vi "GlobalCollectDataRefOperate.vi"(7 "ChannelNbr":u8, 8 "error in (no error)":errorcluster, 9 "DatIn":dbl[][](array[numeric]), 10 "operation":T1, 11 "attributes ref":T2) -> (0 "error out":errorcluster, 1 "SignalDatOut":dbl[][](array[numeric]), 2 "Update":bool)   [LabVIEW 2020, in "DAQ_Base.lvclass"]
doc: "---------------------------------------------------------------\nJKI State Machine Objects™\nhttp://jki.net/state-machine-objects/\nCopyright (C) 2005-2015, JKI <info@jki.net>\nALL RIGHTS RESERVEDJKI State Machine Objects (SMO) 1.0.0.5\nJKI - JKI\nCopyright (c) 2016, JKI"
uses:
  DAQ_Base.lvclass
  utils/ObjectAttributesRef.ctl
  protected/ObjectAttributes.ctl
  protected/DAQSettings.ctl
  protected/SampleSettings.ctl
  protected/AI_ChannelSettings.ctl
  protected/AO_ChannelSettings.ctl
  protected/Cnt_ChannelSettings.ctl
  protected/DataCollector.ctl
  GlobalData_operation.ctl
panel:
  # "For instructions on how to use the JKI State Machine Objects, examples and video tutorials, visit:\nhttp://jki.net/state-machine-objects/\n\nJKI State Machine Objects™\nhttp://jki.net/state-machine-objects/\nCopyright (C) 2005-2015, JKI <info@jki.net>\nALL RIGHTS RESERVED"
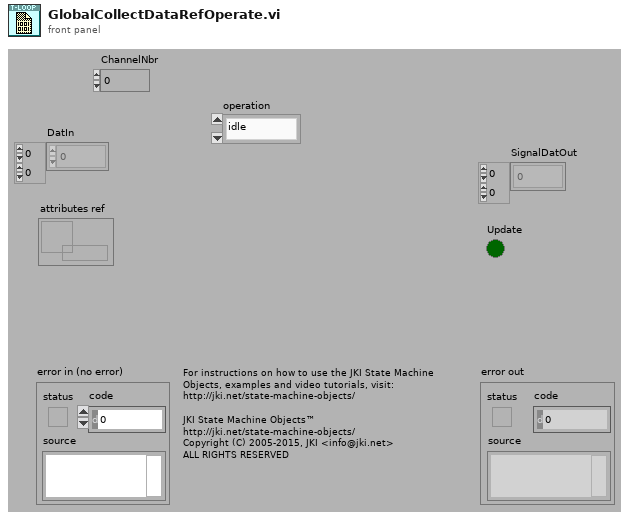
[diagram p1: front panel]
types:
  T1 = typedef "GlobalData_operation.ctl" = enum16{"idle", "read", "write", "clear", "init", "destroy"}
  T2 = typedef "DAQ_Base.lvclass/ObjectAttributesRef.ctl" = refnum<data-value>
  T3 = typedef "DAQ_Base.lvclass/DataCollector.ctl" = cluster{"DataCollectArry":dbl[][], "Update":bool}
  T4 = cluster{"DataCollectArry":dbl[][], "Update":bool}
  T5 = typedef "DAQ_Base.lvclass/ObjectAttributes.ctl" = cluster{"MyAttribute":dbl, "RootPath":path, "DAQSettings":T6, "DaqCollector":cluster{"CollectorChannelEnable":bool[], "CollectDataQueue":refnum<queue>, "ArryDataCollectorChannel":T3[], "RealTimeValues":dbl[]}}
  T6 = typedef "DAQ_Base.lvclass/DAQSettings.ctl" = cluster{"SampleSettings":T7, "AI_ChannelSettings":T8, "AO_ChannelSettings":T10, "Cnt_ChannelSettings":T11}
  T7 = typedef "DAQ_Base.lvclass/SampleSettings.ctl" = cluster{"samples per channel":i32, "SampleRate":dbl, "TansMaxLength":dbl, "ReadTimeOut":dbl, "时钟源":tag}
  T8 = typedef "DAQ_Base.lvclass/AI_ChannelSettings.ctl" = cluster{"AI_SettingsArry":cluster{"DeviceName":tag, "physical channels":tag, "AssignName":string, "输入信号类型":T9, "Max_value":dbl, "Min_value":dbl, "单位":i32, "shunt resistor location":i32, "external shunt resistor value":dbl, "标定系数":cluster{"Scale":dbl, "Offset":dbl}}[]}
  T9 = typedef "AI信号类型.ctl" = i32
  T10 = typedef "DAQ_Base.lvclass/AO_ChannelSettings.ctl" = cluster{"布尔":bool}
  T11 = typedef "DAQ_Base.lvclass/Cnt_ChannelSettings.ctl" = cluster{"Cnt_ChannelSettings":cluster{"类型":enum16{"Linear", "Rotate"}, "CounterNbr":tag, "AssignName":string, "单位":u16, "decoding type":u16, "PPR_DistancePerPulse":dbl, "Initial Position ":dbl, "z index enable":bool, "z index phase":i32, "source":tag}[]}
  T12 = cluster{"DataCollectArry":dbl[][], "Update":bool}[]
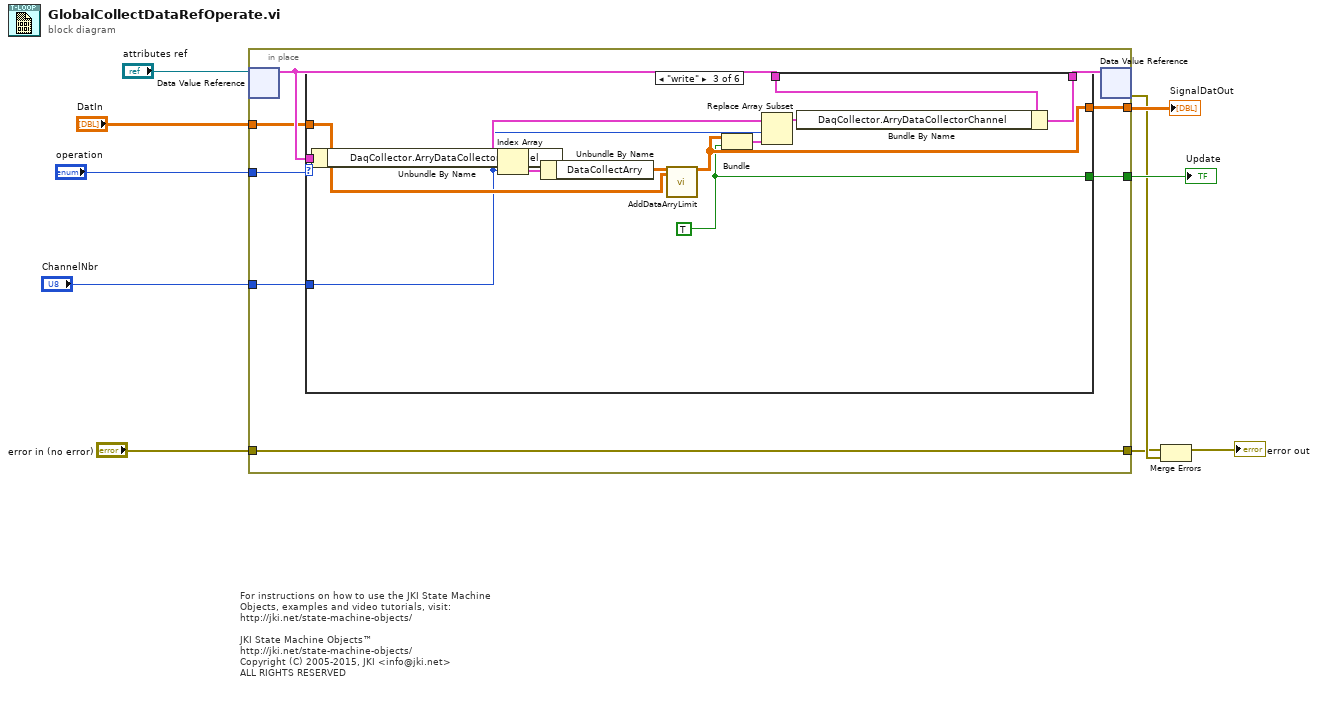
[diagram p0: block diagram]
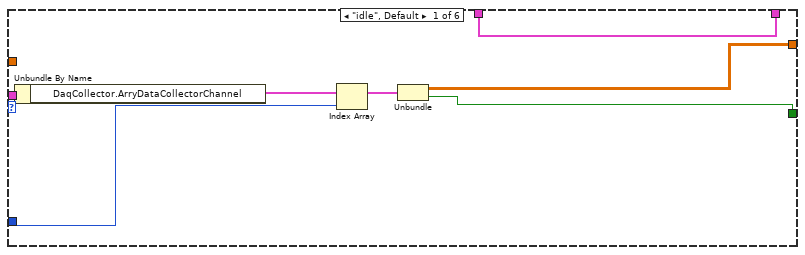
[diagram p2: hidden frame]
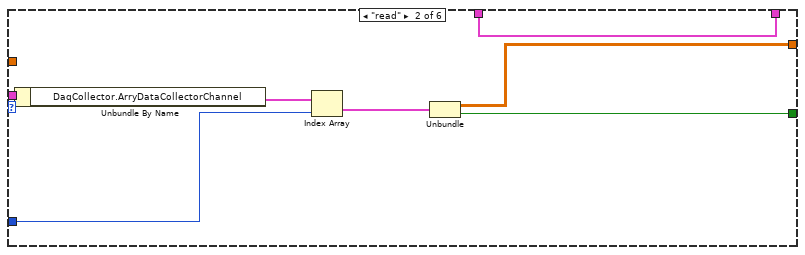
[diagram p3: hidden frame]
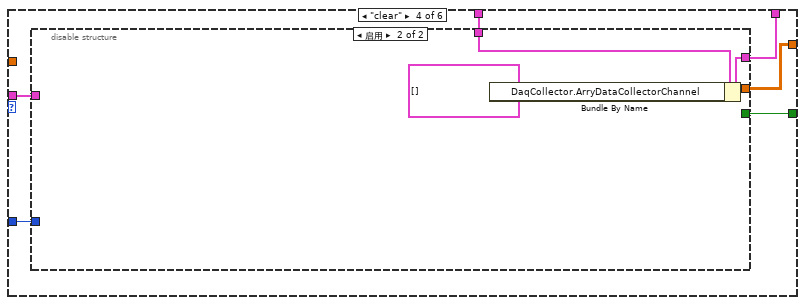
[diagram p4: hidden frame]
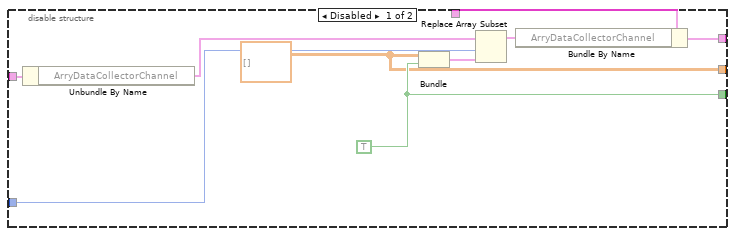
[diagram p5: hidden frame]
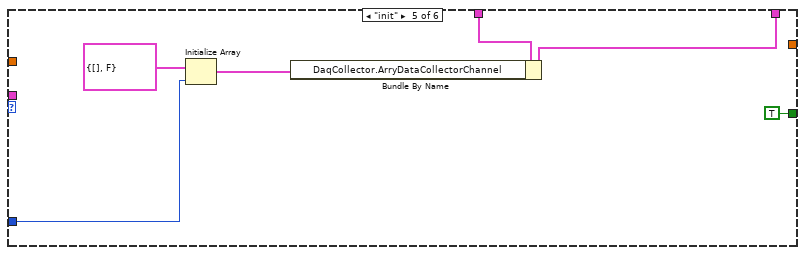
[diagram p6: hidden frame]
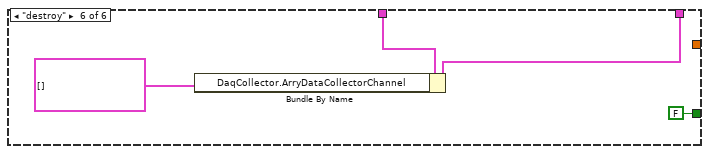
[diagram p7: hidden frame]
diagram:
  # "For instructions on how to use the JKI State Machine Objects, examples and video tutorials, visit:\nhttp://jki.net/state-machine-objects/\n\nJKI State Machine Objects™\nhttp://jki.net/state-machine-objects/\nCopyright (C) 2005-2015, JKI <info@jki.net>\nALL RIGHTS RESERVED"
  n1 = in-place {
    in-place-border: "error in (no error)" -> [w18]
    in-place-border: [w18] -> w1
    in-place-border: [w17] -> w6
    in-place-border: "operation" -> [w16]
    in-place-border: [w15] -> w8
    in-place-border: "DatIn" -> [w12]
    in-place-border: "ChannelNbr" -> [w11]
    n2 = in-place-dvr #1("attributes ref") -> (w14:T5)  [unwired: 1 out]
    n3 = case shown="\"write\"" w16 {
      tunnel: [w20 w27 w38 w45 _ _] -> w17
      tunnel: w14 -> [w22 w30 w44 w50 _ _]
      tunnel: [w19 w26 w37 w47 TRUE ("Update") FALSE ("Update")] -> w15
      tunnel: w14 -> [w25 w32 w43 w49 w68 w72]
      tunnel: [w25 w32 w42 w48 w67 w71] -> w13
      tunnel: w12 -> [_ _ w41 _ _ _]
      tunnel: w11 -> [w21 w29 w35 w46 w64 _]
      frame "idle", Default {
        n4 = Unbundle By Name(w22) -> ("DaqCollector.ArryDataCollectorChannel"=w24:T3[])
        n5 = Index Array(array=w24, index=w21) -> (element=w23:T3)
        n6 = Unbundle(w23) -> ("DataCollectArry"=w20:dbl[][], "Update"=w19:bool)
      }
      frame "read" {
        n7 = Unbundle By Name(w30) -> ("DaqCollector.ArryDataCollectorChannel"=w31:T3[])
        n8 = Index Array(array=w31, index=w29) -> (element=w28:T3)
        n9 = Unbundle(w28) -> ("DataCollectArry"=w27:dbl[][], "Update"=w26:bool)
      }
      frame "write" {
        w37 = TRUE
        n10 = Unbundle By Name(w44) -> ("DaqCollector.ArryDataCollectorChannel"=w36:T3[])
        n11 = Index Array(array=w36, index=w35) -> (element=w40:T3)
        n12 = Unbundle By Name(w40) -> ("DataCollectArry"=w39:dbl[][])
        n13 = call "AddDataArryLimit.vi"("MainDataArryIn"=w39, "SubDataArry"=w41) -> ("输出数组"=w38:dbl[][])  [unwired: 17 in]
        n14 = Bundle("输出数组"=w38, w37) -> (w34:cluster{"输出数组":dbl[][], bool})  [unwired: 1 in]
        n15 = Replace Array Subset(array=w36, new element=w34, index=w35) -> (w33:T3[])
        n16 = Bundle By Name(cluster=w43, "DaqCollector.ArryDataCollectorChannel"=w33) -> (w42:T5)
      }
      frame "clear" {
        n17 = disable-structure shown="启用" {
          disable-tunnel: w50 -> [w59 _]
          disable-tunnel: w49 -> [w58 w62]
          disable-tunnel: [w57 w61] -> w48
          disable-tunnel: [w56 _] -> w47
          disable-tunnel: w46 -> [w54 _]
          disable-tunnel: [w51 _] -> w45
          frame Disabled {
            w51 = dbl[][] [] ("DatIn")
            w56 = TRUE
            n18 = Unbundle By Name(w59) -> ("ArryDataCollectorChannel"=w55:T3[])
            n19 = Bundle("DatIn"=w51, w56) -> (w53:cluster{"DatIn":dbl[][], bool})  [unwired: 1 in]
            n20 = Replace Array Subset(array=w55, new element=w53, index=w54) -> (w52:T3[])
            n21 = Bundle By Name(cluster=w58, "ArryDataCollectorChannel"=w52) -> (w57:T5)
          }
          frame Enabled {
            n22 = Bundle By Name(cluster=w62, "DaqCollector.ArryDataCollectorChannel"=T3[] [] ("ArryDataCollectorChannel")) -> (w61:T5)
          }
        }
      }
      frame "init" {
        n23 = Initialize Array(T4 {"DataCollectArry"=[], "Update"=FALSE} ("DataCollectorChannel"), w64) -> (w63:T12)
        n24 = Bundle By Name(cluster=w68, "DaqCollector.ArryDataCollectorChannel"=w63) -> (w67:T5)
      }
      frame "destroy" {
        n25 = Bundle By Name(cluster=w72, "DaqCollector.ArryDataCollectorChannel"=T3[] [] ("ArryDataCollectorChannel")) -> (w71:T5)
      }
    }
    n26 = in-place-dvr #1(w13) -> (w2:errorcluster)  [unwired: 1 out]
  }
  "Update" <- w8
  "SignalDatOut" <- w6
  n27 = Merge Errors(w1, w2) -> (→"error out":errorcluster)
